vi "Analyze.vi"() -> ()   [LabVIEW 2014]
panel:
  out "Waveform Graph":waveform(dbl)[](graph)
  in  "Log File Path":path
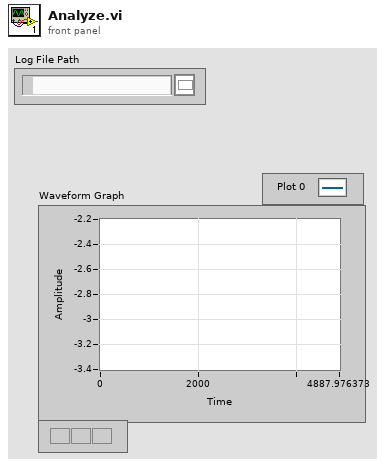
[diagram p1: front panel]
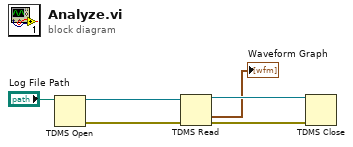
[diagram p0: block diagram]
diagram:
  n1 = TDMS Open(11:"Log File Path") -> (0:w5:errorcluster, 3:w6:refnum<k34>)  [unwired: 6 in]
  n2 = TDMS Read(0:w6, 11:w5) -> (4:w4:refnum<k34>, 10:→"Waveform Graph":waveform(dbl)[], 15:w3:errorcluster)  [unwired: 6 in, 3 out]
  n3 = TDMS Close(8:w3, 11:w4) -> ()  [unwired: 2 out]
